vi "VI Tree.vi"   [LabVIEW 2011, in "Thorlabs_FW102C.lvlib"]
doc: "This is the instrument driver for the <INSTRUMENT NAME>. The VI Tree displays all the user-callable VIs of the instrument driver in an organized table."
uses:
  <instrlib>/Thorlabs_FW102C/Thorlabs_FW102C.lvlib
panel:
  # "(c) 2009 <Enter Company Name Here>.  ALL RIGHTS RESERVED."
  # "SEE DIAGRAM\nFOR VI TREE."
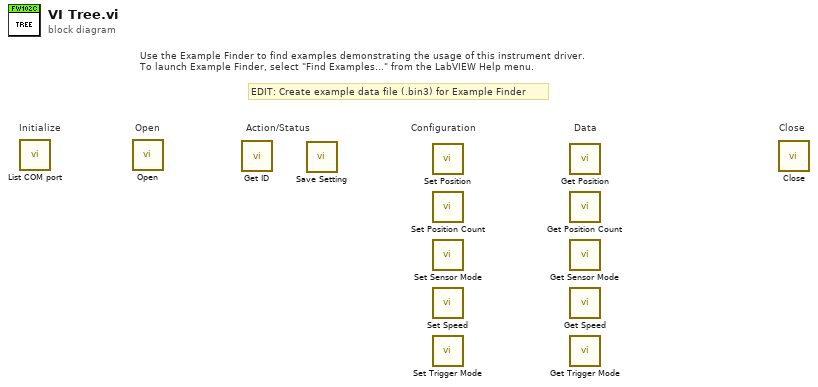
[diagram p0: block diagram]
diagram:
  # "Open"
  # "EDIT: Create example data file (.bin3) for Example Finder"
  # "Use the Example Finder to find examples demonstrating the usage of this instrument driver.\nTo launch Example Finder, select \"Find Examples...\" from the LabVIEW Help menu."
  # "Configuration"
  # "Data"
  # "Action/Status"
  # "Close"
  # "Initialize"
  n1 = call <instrlib>:"List COM port.vi"() -> ()  [unwired: 10 in, 2 out]
  n2 = call <instrlib>:"Open.vi"() -> ()  [unwired: 9 in, 3 out]
  n3 = call <instrlib>:"Get ID.vi"() -> ()  [unwired: 9 in, 3 out]
  n4 = call <instrlib>:"Save Setting.vi"() -> ()  [unwired: 10 in, 2 out]
  n5 = call <instrlib>:"Set Position.vi"() -> ()  [unwired: 10 in, 2 out]
  n6 = call <instrlib>:"Set Position Count.vi"() -> ()  [unwired: 10 in, 2 out]
  n7 = call <instrlib>:"Set Sensor Mode.vi"() -> ()  [unwired: 10 in, 2 out]
  n8 = call <instrlib>:"Set Speed.vi"() -> ()  [unwired: 10 in, 2 out]
  n9 = call <instrlib>:"Set Trigger Mode.vi"() -> ()  [unwired: 10 in, 2 out]
  n10 = call <instrlib>:"Get Position.vi"() -> ()  [unwired: 9 in, 3 out]
  n11 = call <instrlib>:"Get Position Count.vi"() -> ()  [unwired: 9 in, 3 out]
  n12 = call <instrlib>:"Get Sensor Mode.vi"() -> ()  [unwired: 9 in, 3 out]
  n13 = call <instrlib>:"Get Speed.vi"() -> ()  [unwired: 9 in, 3 out]
  n14 = call <instrlib>:"Get Trigger Mode.vi"() -> ()  [unwired: 9 in, 3 out]
  n15 = call <instrlib>:"Close.vi"() -> ()  [unwired: 11 in, 1 out]
